vi "Untitled 5 1.vi"() -> (3 "<JSON>":string="{\n  \"Constant\":{\"Value\":21},\n  \"Fn. Gen\":{\n    \"Min Value\":-10,\n    \"Max Value\":10,\n    \"Duty Cycle (%)\":50,\n    \"Signal Type\":2,\n    \"Cycle Number\":10,\n    \"Phase (degrees)\":0\n  },\n  \"Formula\":{\n    \"formula\":\"10 * sin(1 * 3.141592653 * t)\",\n    \"formula length (nm)\":1,\n    \"formula resolution (nm)\":0.01\n  },\n  \"Ramp\":{\"Start\":0,\"End\":10}\n}")   [LabVIEW 2019]
uses:
  subVIs/typedefs/Schedule Types/Schedule--Constant.ctl
  subVIs/typedefs/Schedule Types/Schedule--Function Generator.ctl
  subVIs/typedefs/Schedule Types/Schedule--Formula.ctl
  subVIs/typedefs/Schedule Types/Schedule--Ramp.ctl
  e82f576e-e58b-432b-9cb2-f230db120042.vi
  <vilib>/JDP Science/JSONtext/Variant to JSON Text.vi
  <vilib>/JDP Science/JSONtext/LVClass Serializer/JSONtext LVClass Serializer.lvclass
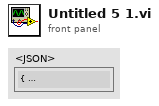
[diagram p1: front panel]
types:
  T1 = typedef "Schedule--Constant.ctl" = cluster{"Value":dbl}
  T2 = typedef "Schedule--Function Generator.ctl" = cluster{"Min Value":dbl, "Max Value":dbl, "Duty Cycle (%)":dbl, "Signal Type":u16, "Cycle Number":dbl, "Phase (degrees)":dbl}
  T3 = typedef "Schedule--Formula.ctl" = cluster{"formula":string, "formula length (nm)":dbl, "formula resolution (nm)":dbl}
  T4 = typedef "Schedule--Ramp.ctl" = cluster{"Start":dbl, "End":dbl}
  T5 = cluster{"Constant":T1, "Fn. Gen":T2, "Formula":T3, "Ramp":T4}
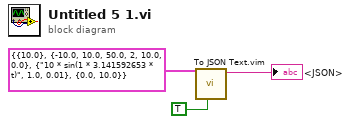
[diagram p0: block diagram]
diagram:
  n1 = call "To JSON Text.vim"("Pretty Print?"=TRUE, "Anything"=T5 {"Constant"={"Value"=10.0}, "Fn. Gen"={"Min Value"=-10.0, "Max Value"=10.0, "Duty Cycle (%)"=50.0, "Signal Type"=2, "Cycle Number"=10.0, "Phase (degrees)"=0.0}, "Formula"={"formula"="10 * sin(1 * 3.141592653 * t)", "formula length (nm)"=1.0, "formula resolution (nm)"=0.01}, "Ramp"={"Start"=0.0, "End"=10.0}}) -> ("<JSON>"=→"<JSON>":string)  [unwired: 8 in, 1 out]
